vi "DateTimeToString.vi"(8 "error in":errorcluster, 10 "current time":timestamp, 11 "include Time?":bool) -> (0 "error out":errorcluster, 2 "date string":string)   [LabVIEW 2019, in "ByteGSWebAPI.lvlib" / "ByteGSAPIBase.lvclass"]
doc: "Cast a date from Labview format to String, with the option to include the time"
uses:
  ByteGSAPIBase.lvclass
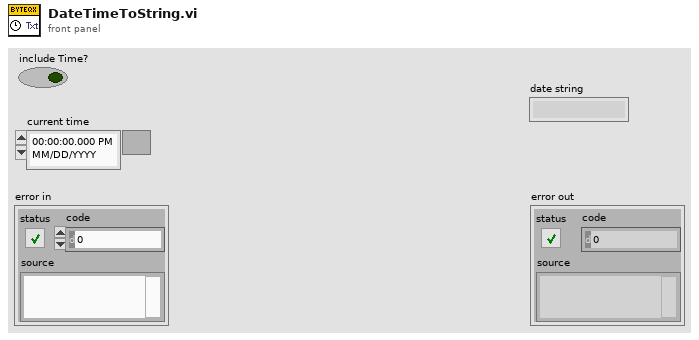
[diagram p1: front panel]
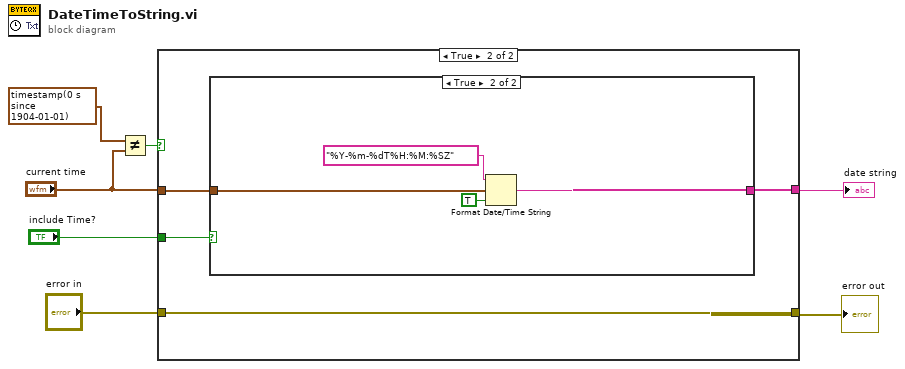
[diagram p0: block diagram]
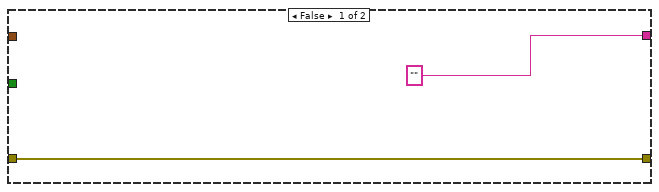
[diagram p2: hidden frame]
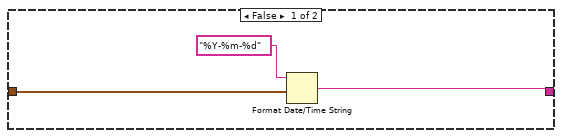
[diagram p3: hidden frame]
diagram:
  n1 = Not Equal?(x=timestamp(0 s since 1904-01-01) ("current time 2"), y="current time") -> (x != y?=w5:bool)
  n2 = case shown="True" w5 {
    tunnel: ["" w11] -> w7
    tunnel: "current time" -> [_ w12]
    tunnel: "error in" -> [w8 w13]
    tunnel: [w8 w13] -> w2
    tunnel: "include Time?" -> [_ w10]
    frame False {
    }
    frame True {
      n3 = case shown="True" w10 {
        tunnel: w12 -> [w15 w19]
        tunnel: [w14 w18] -> w11
        frame False {
          n4 = Format Date/Time String(time format string (%c)="%Y-%m-%d", seconds (now)=w15) -> (date/time string=w14:string)  [unwired: 1 in]
        }
        frame True {
          n5 = Format Date/Time String(time format string (%c)="%Y-%m-%dT%H:%M:%SZ", seconds (now)=w19, UTC format=TRUE) -> (date/time string=w18:string)
        }
      }
    }
  }
  "date string" <- w7
  "error out" <- w2
